vi "PlugIn_Backpack.vi"(10 "Console":string) -> ()   [LabVIEW 2021]
panel:
  in  "stop":bool
  out "Spike":string
  out "Dongle":string
  in  "Send to backpack":string
  in  "Send":bool
  in  "Clear":bool
  in  "Ctrl C":bool
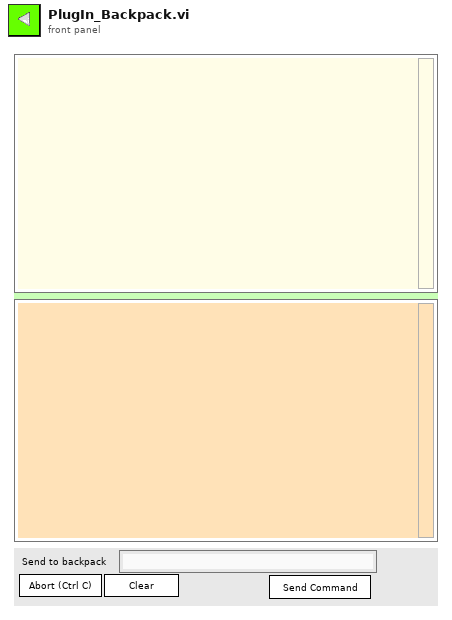
[diagram p1: front panel]
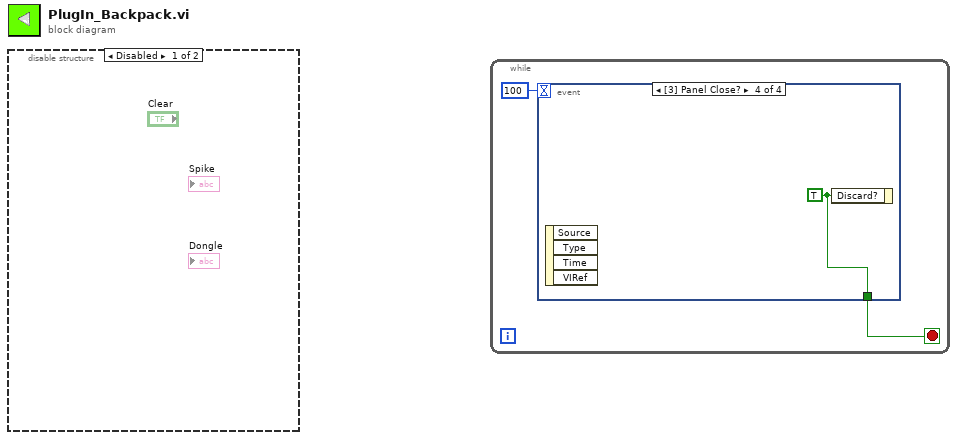
[diagram p0: block diagram]
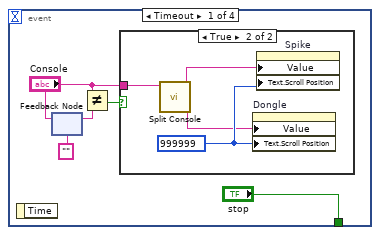
[diagram p2: hidden frame]
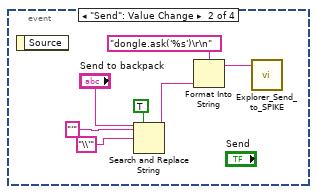
[diagram p4: hidden frame]
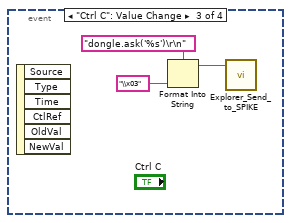
[diagram p5: hidden frame]
diagram:
  n1 = disable-structure shown="Disabled" {
    frame Disabled {
    }
    frame Enabled {
    }
  }
  n2 = while {
    stop <- w2 stop-if-true
    n3 = event shown="[3] Panel Close?" {
      selector: _ -> [_ _ _ _]
      dyn-events: _ -> [_ _ _ _]
      timeout: 100 -> [_ _ _ _]
      tunnel: ["stop" _ _ w22] -> w2
      event Timeout {
        n4 = event-data() -> ()  [unwired: 1 in, 1 out]
        n5 = feedback-in #1("Console") -> ()
        n6 = feedback #1("" ("Console")) -> (w6:string)
        n7 = Not Equal?(x="Console", y=w6) -> (x != y?=w3:bool)
        n8 = case shown="True" w3 {
          tunnel: "Console" -> [_ w11]
          frame False {
          }
          frame True {
            w10 = u32 999999 ("Text.Selection:End")
            n9 = call "Split Console.vi"("Console"=w11) -> ("Dongle"=w8:string, "Spike"=w9:string)  [unwired: 9 in]
            n10 = property on="Dongle" class="Str"("Value"=w8, "Text.Scroll Position"=w10) -> ()  [unwired: 2 in, 2 out]
            n11 = property on="Spike" class="Str"("Value"=w9, "Text.Scroll Position"=w10) -> ()  [unwired: 2 in, 2 out]
          }
        }
      }
      event "Send": Value Change {
        n12 = event-data() -> ()  [unwired: 1 in, 1 out]
        n13 = Search and Replace String(replace all?=TRUE ("replace all? (F)"), input string="Send to backpack", search string="'" ("string"), replace string="\\'" ("string")) -> (result string=w14:string)  [unwired: 4 in, 3 out]
        n14 = Format Into String(format string="dongle.ask('%s')\r\n" ("string"), w14) -> (resulting string=w18:string)  [unwired: 2 in, 1 out]
        n15 = call "Explorer_Send_to_SPIKE.vi"("python"=w18) -> ()  [unwired: 10 in, 1 out]
      }
      event "Ctrl C": Value Change {
        n16 = event-data() -> ()  [unwired: 1 in, 6 out]
        n17 = Format Into String(format string="dongle.ask('%s')\r\n" ("string"), "\\x03" ("Send to backpack 2")) -> (resulting string=w20:string)  [unwired: 2 in, 1 out]
        n18 = call "Explorer_Send_to_SPIKE.vi"("python"=w20) -> ()  [unwired: 10 in, 1 out]
      }
      event Panel Close? {
        w22 = TRUE ("Discard?")
        n19 = event-data() -> ()  [unwired: 1 in, 4 out]
        n20 = event-data("Discard?"=w22) -> ()  [unwired: 1 in, 1 out]
      }
    }
  }
